vi "blink.vi"(11 "Array":dbl[](array[numeric])) -> (3 "Glitter":bool)   [LabVIEW 2014]
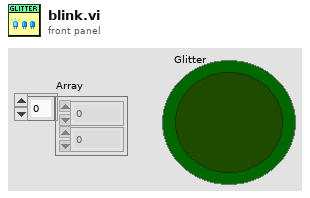
[diagram p1: front panel]
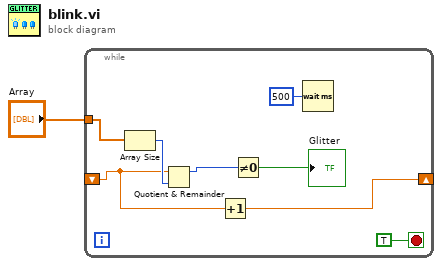
[diagram p0: block diagram]
diagram:
  n1 = while {
    shift-right: [w2] -> _
    shift-left: _ -> [w3]
    tunnel: "Array" -> [w9]
    stop <- TRUE stop-if-true
    n2 = Array Size(array=w9) -> (size(s)=w8:i32)
    n3 = Quotient & Remainder(x=w3, y=w8) -> (x-y*floor(x/y)=w7:i32)  [unwired: 1 out]
    n4 = Increment(x=w3) -> (x+1=w2:dbl)
    n5 = Not Equal To 0?(x=w7) -> (x != 0?=→"Glitter":bool)
    n6 = Wait (ms)(milliseconds to wait=u32 500) -> ()  [unwired: 1 out]
  }
